vi "Compute DistanceToTarget.vi"(7 "left?":bool, 8 "Y Image Resolution":i32, 9 "X Image Resolution":i32, 10 "Vertical Strip":T1, 11 "Camera Type":enum16{"206", "1011", "1013"}(ring)) -> (1 "Angle":dbl, 2 "Target Center (-1 to 1)":cluster{"X":dbl, "Y":dbl}, 3 "Distance (ft)":dbl)   [LabVIEW 2015]
doc: "Using the camera lens information and the real world size of the target, use trig and ratios to determine the distance to the target. Also returns the location relative to the image center in a (-1 , 1) coordinate system that may be useful for steering the robot."
panel:
  in  "Camera view angles":dbl[](array[numeric])=[41.7, 37.4, 49.0]
  # "Axis 206\nAxis M1011\nAxis M1013"
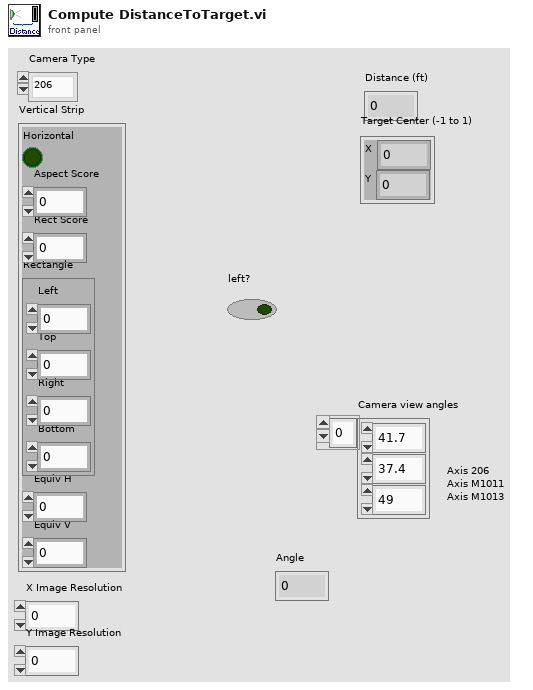
[diagram p1: front panel]
types:
  T1 = cluster{"Horizontal":bool, "Aspect Score":dbl, "Rect Score":dbl, "Rectangle":cluster{"Left":dbl, "Top":dbl, "Right":dbl, "Bottom":dbl}, "Equiv H":dbl, "Equiv V":dbl}
  T2 = cluster{"X Image Resolution":i32, "Y Image Resolution":i32}
  T3 = cluster{"X Image Resolution":dbl, "Y Image Resolution":dbl}
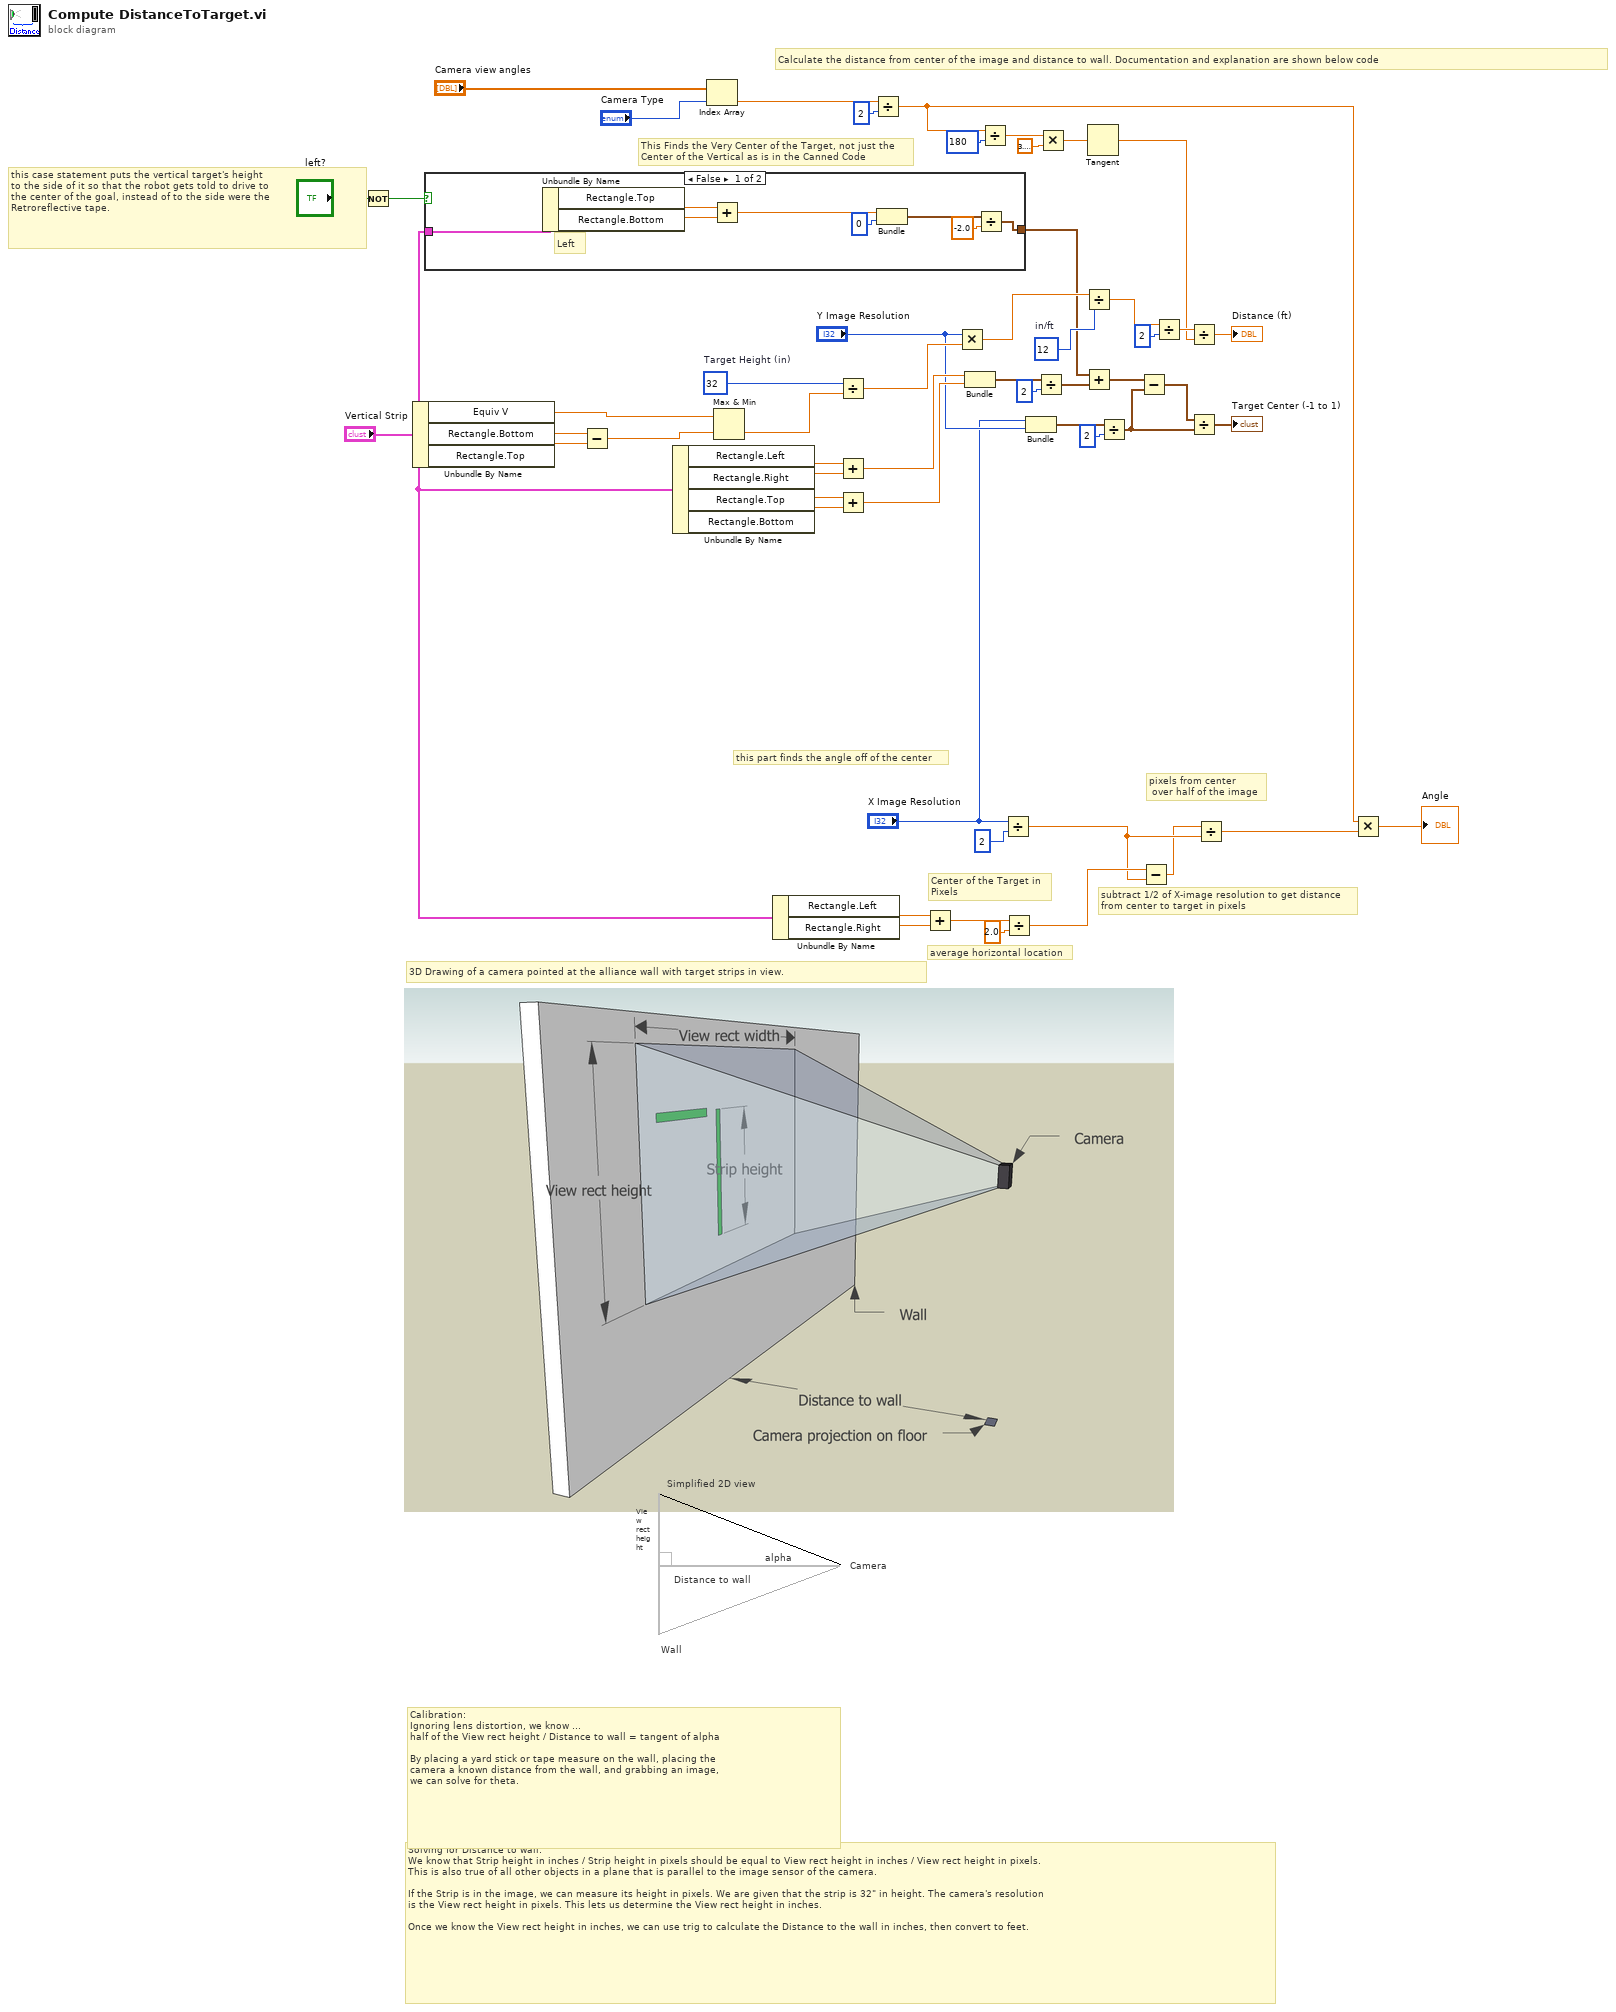
[diagram p0: block diagram]
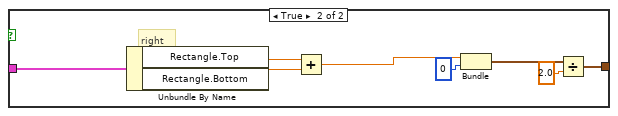
[diagram p2: hidden frame]
diagram:
  w24 = 12  # in/ft
  w29 = 32  # Target Height (in)
  # "pixels from center\n over half of the image"
  # "Center of the Target in \nPixels"
  # "subtract 1/2 of X-image resolution to get distance\nfrom center to target in pixels"
  # "average horizontal location"
  # "this part finds the angle off of the center"
  # "This Finds the Very Center of the Target, not just the \nCenter of the Vertical as is in the Canned Code"
  # "this case statement puts the vertical target's height\nto the side of it so that the robot gets told to drive to\nthe center of the goal, instead of to the side were the\nRetroreflective tape."
  # "Wall"
  # "Camera"
  # "Simplified 2D view"
  # "Solving for Distance to wall:\nWe know that Strip height in inches / Strip height in pixels should be equal to View rect height in inches / View rect height in pixels.\nThis is also true of all other objects in a plane that is parallel to the image sensor of the camera.\n\nIf the Strip is in the image, we can measure its height in pixels. We are given that the strip is 32\" in height. The camera's resolution\nis the View rect height in pixels. This lets us determine the View rect height in inches.\n\nOnce we know the View rect height in inches, we can use trig to calculate the Distance to the wall in inches, then convert to feet."
  # "3D Drawing of a camera pointed at the alliance wall with target strips in view."
  # "Distance to wall"
  # "View rect height"
  # "alpha"
  # "Calibration:\nIgnoring lens distortion, we know ...\nhalf of the View rect height / Distance to wall = tangent of alpha\n\nBy placing a yard stick or tape measure on the wall, placing the\ncamera a known distance from the wall, and grabbing an image,\nwe can solve for theta."
  # "Calculate the distance from center of the image and distance to wall. Documentation and explanation are shown below code"
  n1 = Not(x="left?") -> (.not. x?=w14:bool)
  n2 = Unbundle By Name("Vertical Strip") -> ("Equiv V"=w31:dbl, "Rectangle.Bottom"=w46:dbl, "Rectangle.Top"=w45:dbl)
  n3 = case shown="False" w14 {
    tunnel: "Vertical Strip" -> [w56 w63]
    tunnel: [w55 w66] -> w18
    frame False {
      # "Left"
      n4 = Unbundle By Name(w56) -> ("Rectangle.Top"=w62:dbl, "Rectangle.Bottom"=w61:dbl)
      n5 = Add(x=w62, y=w61) -> (x+y=w60:dbl)
      n6 = Bundle(w60, 0) -> (w57:cluster{dbl, i32})  [unwired: 1 in]
      n7 = Divide(x=w57, y=-2.0) -> (x/y=w55:cluster{dbl, dbl})
    }
    frame True {
      # "right"
      n8 = Unbundle By Name(w63) -> ("Rectangle.Top"=w70:dbl, "Rectangle.Bottom"=w69:dbl)
      n9 = Add(x=w70, y=w69) -> (x+y=w68:dbl)
      n10 = Bundle(w68, 0) -> (w64:cluster{dbl, i32})  [unwired: 1 in]
      n11 = Divide(x=w64, y=2.0) -> (x/y=w66:cluster{dbl, dbl})
    }
  }
  n12 = Subtract(x=w46, y=w45) -> (x-y=w30:dbl)
  n13 = Unbundle By Name("Vertical Strip") -> ("Rectangle.Left"=w41:dbl, "Rectangle.Right"=w42:dbl, "Rectangle.Top"=w44:dbl, "Rectangle.Bottom"=w43:dbl)
  n14 = Index Array(array="Camera view angles", index="Camera Type") -> (element=w51:dbl)
  n15 = Max & Min(x=w31, y=w30) -> (min(x,y)=w28:dbl)  [unwired: 1 out]
  n16 = Unbundle By Name("Vertical Strip") -> ("Rectangle.Left"=w12:dbl, "Rectangle.Right"=w11:dbl)
  n17 = Divide(x=w29, y=w28) -> (x/y=w27:dbl)
  n18 = Add(x=w41, y=w42) -> (x+y=w39:dbl)
  n19 = Add(x=w44, y=w43) -> (x+y=w38:dbl)
  n20 = Divide(x=w51, y=2) -> (x/y=w4:dbl)
  n21 = Add(x=w12, y=w11) -> (x+y=w10:dbl)
  n22 = Multiply(x="Y Image Resolution", y=w27) -> (x*y=w25:dbl)
  n23 = Bundle(w39, w38) -> (w35:cluster{dbl, dbl})  [unwired: 1 in]
  n24 = Divide(x=w4, y=180) -> (x/y=w48:dbl)
  n25 = Divide(x="X Image Resolution", y=2) -> (x/y=w2:dbl)
  n26 = Divide(x=w10, y=2.0) -> (x/y=w6:dbl)
  n27 = Bundle("X Image Resolution"="X Image Resolution", "Y Image Resolution"="Y Image Resolution") -> (w37:T2)  [unwired: 1 in]
  n28 = Divide(x=w35, y=2) -> (x/y=w17:cluster{dbl, dbl})
  n29 = Multiply(x=w48, y=3.141592653589793) -> (x*y=w49:dbl)
  n30 = Divide(x=w25, y=w24) -> (x/y=w23:dbl)
  n31 = Add(x=w18, y=w17) -> (x+y=w16:cluster{dbl, dbl})
  n32 = Tangent(1:w49) -> (0:w20:dbl)
  n33 = Divide(x=w37, y=2) -> (x/y=w33:T3)
  n34 = Subtract(x=w16, y=w33) -> (x-y=w34:cluster{dbl, dbl})
  n35 = Subtract(x=w6, y=w2) -> (x-y=w1:dbl)
  n36 = Divide(x=w23, y=2) -> (x/y=w21:dbl)
  n37 = Divide(x=w21, y=w20) -> (x/y=→"Distance (ft)":dbl)
  n38 = Divide(x=w34, y=w33) -> (x/y=→"Target Center (-1 to 1)":cluster{dbl, dbl})
  n39 = Divide(x=w1, y=w2) -> (x/y=w5:dbl)
  n40 = Multiply(x=w4, y=w5) -> (x*y=→"Angle":dbl)
